vi "EmergencyPowerStateController.vi"   [LabVIEW 2019]
uses:
  dsinstructions.vi
  outputs.vi
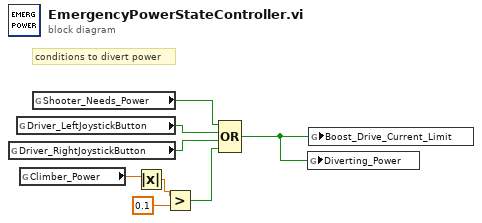
[diagram p0: block diagram]
diagram:
  # "conditions to divert power"
  n1 = global read "dsinstructions.vi" "Driver_RightJoystickButton"() -> (w8:bool)
  n2 = global read "dsinstructions.vi" "Driver_LeftJoystickButton"() -> (w7:bool)
  n3 = global read "outputs.vi" "Climber_Power"() -> (w5:dbl)
  n4 = global read "outputs.vi" "Shooter_Needs_Power"() -> (w1:bool)
  n5 = Absolute Value(x=w5) -> (abs(x)=w2:dbl)
  n6 = Greater?(x=w2, y=0.1) -> (0:w3:bool)
  n7 = Compound Arithmetic op=OR(w1, w7, w8, w3) -> (w6:bool)
  n8 = global write "outputs.vi" "Diverting_Power"(w6) -> ()
  n9 = global write "outputs.vi" "Boost_Drive_Current_Limit"(w6) -> ()
